vi "Can_SendData.vi"(4 "Seq?":bool, 6 "Data":T1=[{"identifier"=1715, "payload"=[2, 16, 3, 255, 255, 255, 255, 255], "Send?"=FALSE, "Note"="", "Delays"=100, "Seq"=0}] {"payload" format="%02x"; "identifier" format="%x"}, 7 "mode":enum16{"Init", "Send"}(ring)=enum."Send", 8 "error in (no error)":errorcluster, 9 "Interface:Baud Rate":u32=250000, 10 "cluster (:memory:)":refnum<k21>="Z177TEST", 11 "interface":refnum<k21>="CAN2") -> (0 "error":errorcluster)   [LabVIEW 2015]
uses:
  Crl/Can_DataType.ctl
  <vilib>/xnet/xnet.llb/XNET Frame CAN.ctl
  <vilib>/xnet/xnet.llb/XNET Frame Type CAN.ctl
  <vilib>/xnet/xnet.llb/XNET Create Session (Frame Output Stream).vi
  <vilib>/xnet/xnet.llb/XNET Write (Frame CAN).vi
  <resource>/objmgr/xnet.rc
panel:
  # "ms"
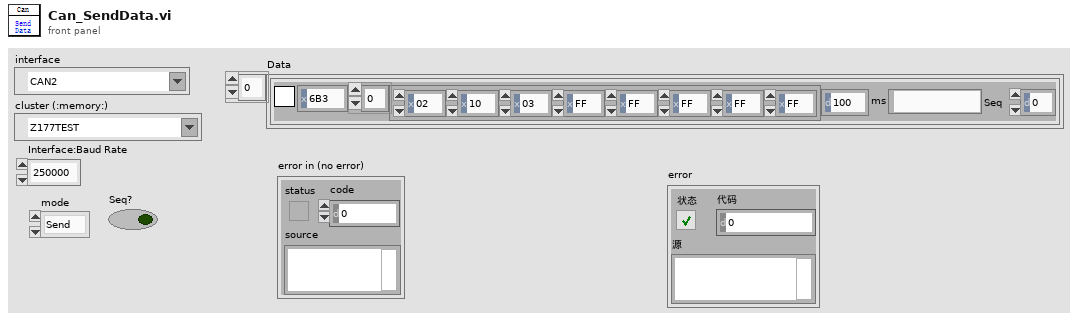
[diagram p1: front panel]
types:
  T1 = typedef "Can_DataType.ctl" = cluster{"identifier":u32, "payload":u8[], "Send?":bool, "Note":string, "Delays":u32, "Seq":i32}[]
  T2 = cluster{"error":errorcluster, "session":refnum<k21>}
  T3 = typedef "XNET Frame CAN.ctl" = cluster{"timestamp":timestamp, "payload":u8[], "identifier":u32, "type":T4, "extended?":bool, "echo?":bool}
  T4 = typedef "XNET Frame Type CAN.ctl" = u8
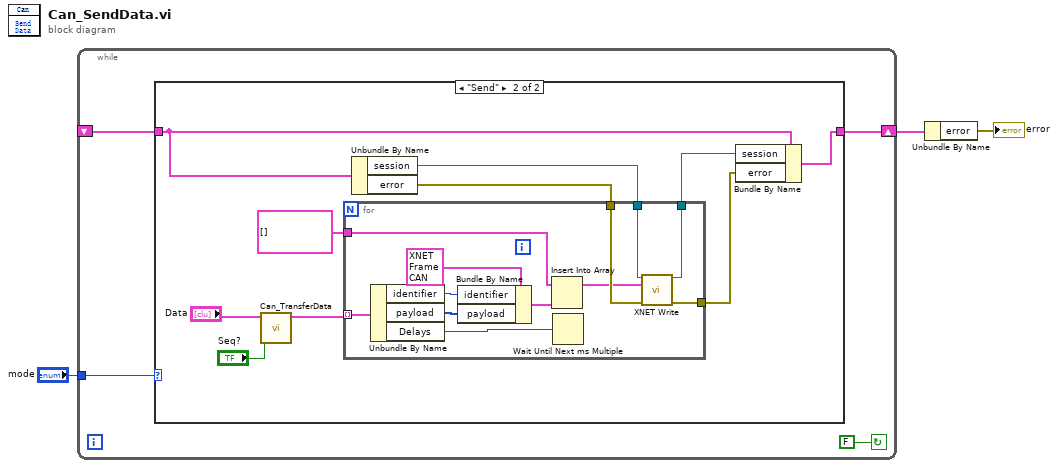
[diagram p0: block diagram]
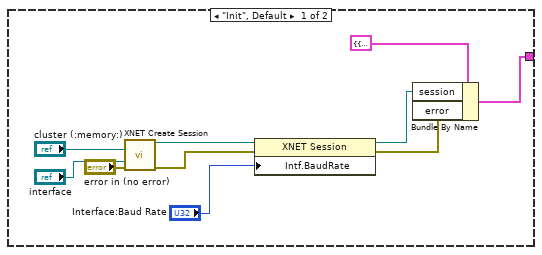
[diagram p2: hidden frame]
diagram:
  n1 = while {
    shift-right: [w4] -> w2
    shift-left: _ -> [w6]
    tunnel: "mode" -> [w7]
    stop <- FALSE continue-if-true
    n2 = case shown="\"Send\"" w7 {
      tunnel: [w10 w22] -> w4
      tunnel: w6 -> [_ w26]
      frame "Init", Default {
        n3 = call-poly <vilib>:"XNET Create Session.vi"("cluster (:memory:)"="cluster (:memory:)", "interface"="interface", "error in (no error)"="error in (no error)") -> ("session out"=w15:refnum<k21>, "error out"=w17:errorcluster)  [unwired: 11 out]
        n4 = property class="XNET Session"(reference=w15, error in=w17, "Intf.BaudRate"="Interface:Baud Rate") -> (reference out=w12:refnum<k21>, error out=w11:errorcluster)
        n5 = Bundle By Name(cluster=T2 {"error"={"status"=FALSE, "code"=0, "source"=""}, "session"=""}, "session"=w12, "error"=w11) -> (w10:T2)
      }
      frame "Send" {
        n6 = call "Can_TransferData.vi"("Seq?"="Seq?", "Data"="Data") -> ("Data"=w19:T1)  [unwired: 9 in]
        n7 = Unbundle By Name(w26) -> ("session"=w27:refnum<k21>, "error"=w24:errorcluster)
        n8 = for {
          tunnel: w19 -> [w34] mode=indexing
          tunnel: T3[] [] ("data") -> [w37]
          tunnel: w27 -> [w33]
          tunnel: w24 -> [w32]
          tunnel: [w30] -> w25
          tunnel: [w29] -> w23
          n9 = Unbundle By Name(w34) -> ("identifier"=w38:u32, "payload"=w39:u8[], "Delays"=w28:u32)
          n10 = Bundle By Name(cluster=T3 {"timestamp"=timestamp(0 s since 1904-01-01), "payload"=[], "identifier"=0, "type"=0, "extended?"=FALSE, "echo?"=FALSE} ("CAN frame"), "identifier"=w38, "payload"=w39) -> (w35:T3)
          n11 = Insert Into Array(array=w37, new element=w35) -> (w31:T3[])  [unwired: 1 in]
          n12 = Wait Until Next ms Multiple(millisecond multiple=w28) -> ()  [unwired: 1 out]
          n13 = call-poly <vilib>:"XNET Write.vi"("session in"=w33, "data"=w31, "error in (no error)"=w32) -> ("session out"=w30:refnum<k21>, "error out"=w29:errorcluster)  [unwired: 11 out]
        }
        n14 = Bundle By Name(cluster=w26, "session"=w25, "error"=w23) -> (w22:T2)
      }
    }
  }
  n15 = Unbundle By Name(w2) -> ("error"=→"error":errorcluster)
